vi "LVClass_CameraSet Get Actions List.vi"(0 "CameraSet in":refnum<class "CameraSet.lvclass">, 11 "error in (no error)":errorcluster) -> (4 "CameraSet out":refnum<class "CameraSet.lvclass">, 6 "Actions list":string[](array[string]), 15 "error out":errorcluster)   [LabVIEW 2020, in "CameraSet.lvclass"]
uses:
  CameraSet.lvclass
  CameraSet.lvclass/CameraSet.ctl
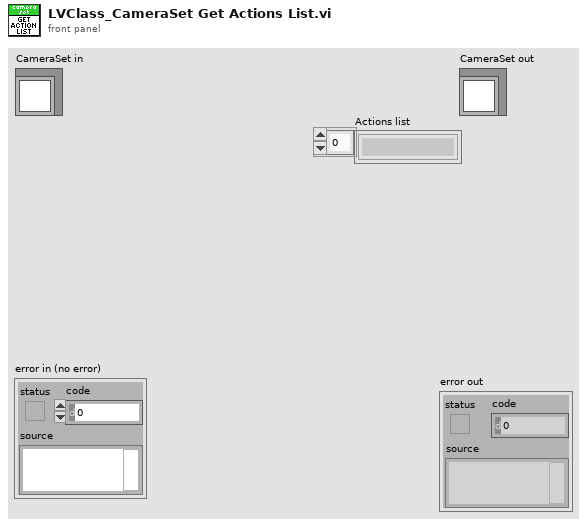
[diagram p1: front panel]
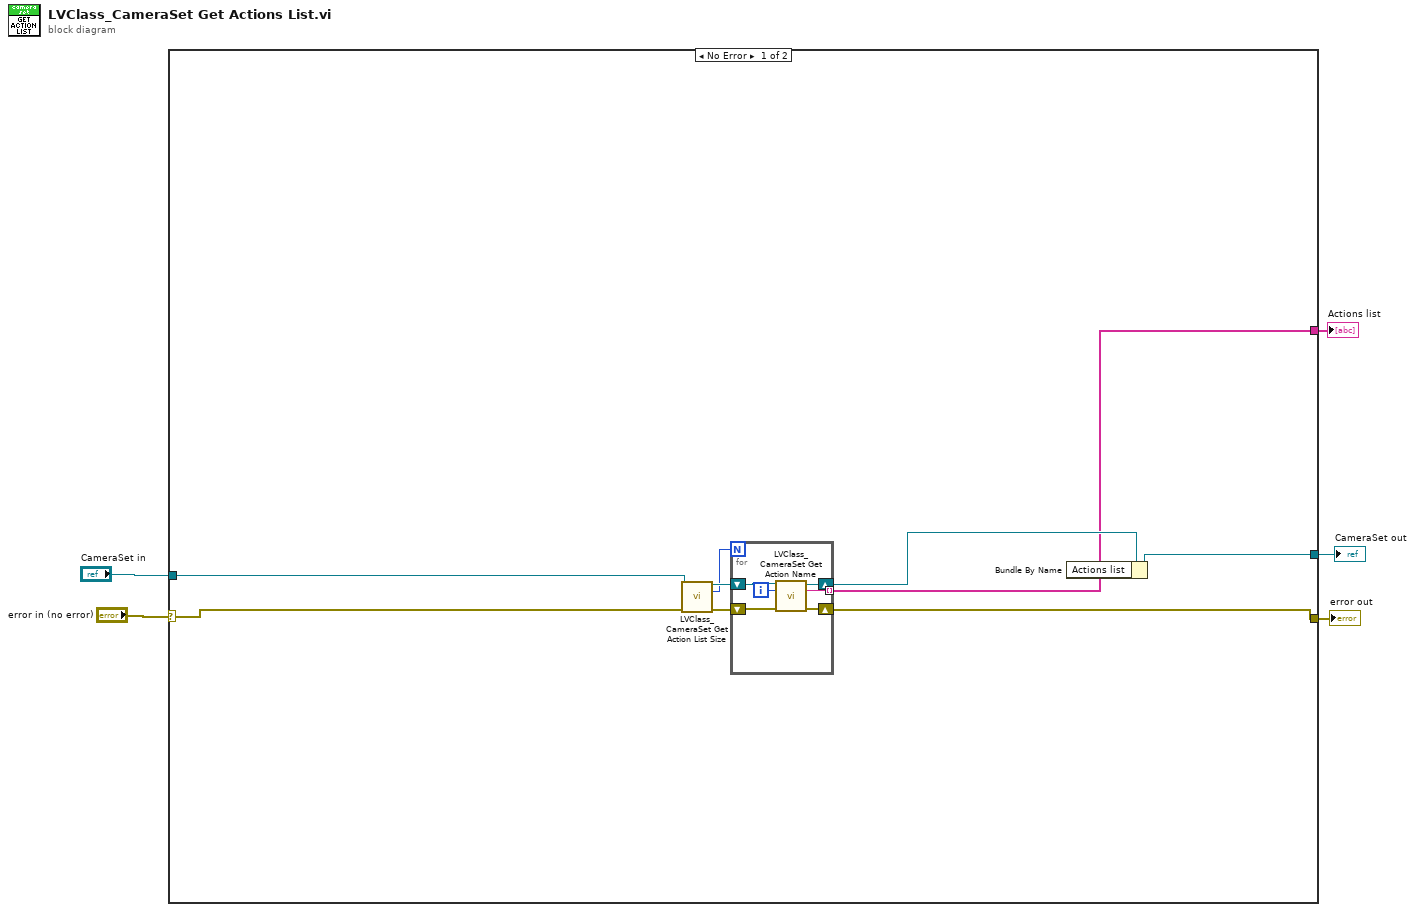
[diagram p0: block diagram]
diagram:
  n1 = case shown="No Error" "error in (no error)" {
    selector: "error in (no error)" -> [w10 w22]
    tunnel: [w9 w22] -> w4
    tunnel: [w7 w21] -> w2
    tunnel: "CameraSet in" -> [w11 w21]
    tunnel: [w6 _] -> w1
    frame No Error {
      n2 = call "LVClass_CameraSet Get Action List Size.vi"("CameraSet.lvclass"=w11, "error in (no error)"=w10) -> ("CameraSet.lvclass"=w13:refnum<class "CameraSet.lvclass">, "size"=w12:i32, "error out"=w14:errorcluster)  [unwired: 11 in]
      n3 = for {
        N: w12 -> [_]
        shift-right: [w20] -> w8
        shift-left: w13 -> [w19]
        shift-right: [w16] -> w9
        shift-left: w14 -> [w17]
        tunnel: [w15] -> w6 mode=indexing
        i -> [w18]
        n4 = call "LVClass_CameraSet Get Action Name.vi"("CameraSet.lvclass"=w19, "index"=w18, "error in (no error)"=w17) -> ("CameraSet.lvclass"=w20:refnum<class "CameraSet.lvclass">, "action_name"=w15:string, "error out"=w16:errorcluster)  [unwired: 10 in]
      }
      n5 = Bundle By Name(cluster=w8, "Actions list"=w6) -> (w7:refnum<class "CameraSet.lvclass">)
    }
    frame Error {
    }
  }
  "error out" <- w4
  "CameraSet out" <- w2
  "Actions list" <- w1
